vi "Reset Acyclic Channels.vi"(8 "error in (no error)":errorcluster, 11 "Single Board Loopback in":refnum<class "Single Board Loopback.lvclass">) -> (0 "error out":errorcluster, 3 "Single Board Loopback out":refnum<class "Single Board Loopback.lvclass">)   [LabVIEW 2020]
uses:
  Single Board Loopback/Single Board Loopback.lvclass
  C:/Users/nitest/Desktop/Git 2020/niveristand-custom-device-testing-tools/VeriStandTestCase/VeriStandTestCase.lvclass
  1e32ca70-98be-4c49-9a55-e48adc1a34b6.vi
  <vilib>/NI VeriStand/Execution/Workspace/NI VeriStand - Set Multiple Channel Values.vi
  niveristand-custom-device-testing-tools/VeriStandTestUtilities/VeriStandTestUtilities.lvlib
  <vilib>/NI VeriStand/Execution/Workspace/NI_VS Workspace ExecutionAPI.lvlib
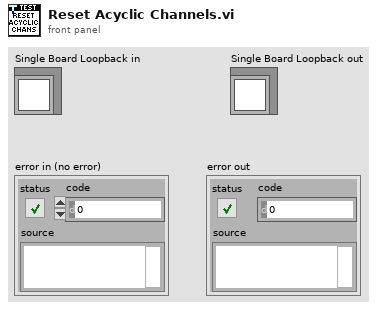
[diagram p1: front panel]
types:
  T1 = typedef "NI_VS Workspace ExecutionAPI.lvlib/WorkspaceAPI.ctl" = refnum<k24>
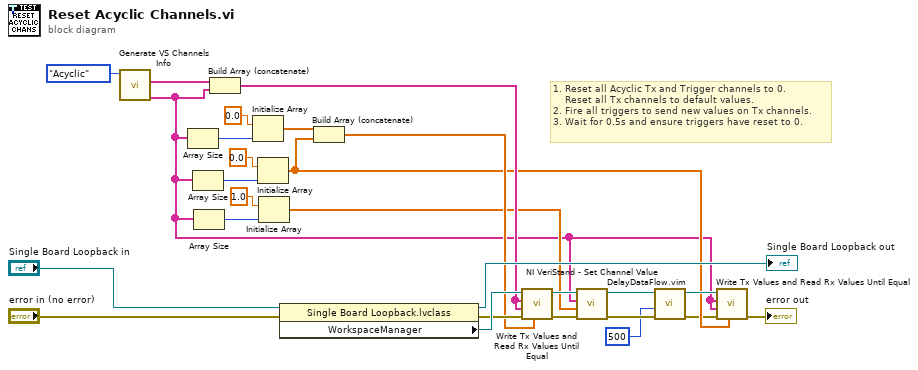
[diagram p0: block diagram]
diagram:
  # "1. Reset all Acyclic Tx and Trigger channels to 0.\n    Reset all Tx channels to default values.\n2. Fire all triggers to send new values on Tx channels.\n3. Wait for 0.5s and ensure triggers have reset to 0."
  n1 = call "Generate VS Channels Info.vi"("Transfer Type"=enum16{"Acyclic", "Scheduled"}."Acyclic") -> ("Tx Trigger Channels Array"=w1:string[], "Tx Channels Array"=w23:string[])  [unwired: 6 in, 3 out]
  n2 = Array Size(array=w1) -> (size(s)=w3:i32)
  n3 = Array Size(array=w1) -> (size(s)=w22:i32)
  n4 = Array Size(array=w1) -> (size(s)=w13:i32)
  n5 = Build Array (concatenate)(w23, w1) -> (w19:string[])
  n6 = Initialize Array(0.0 ("element"), w3) -> (w2:dbl[])
  n7 = Initialize Array(0.0 ("element"), w22) -> (w10:dbl[])
  n8 = Initialize Array(1.0 ("element"), w13) -> (w11:dbl[])
  n9 = property class="Single Board Loopback.lvclass"(reference="Single Board Loopback in", error in="error in (no error)") -> (reference out=→"Single Board Loopback out":refnum<class "Single Board Loopback.lvclass">, error out=w20:errorcluster, "WorkspaceManager"=w24:T1)
  n10 = Build Array (concatenate)(w2, w10) -> (w18:dbl[])
  n11 = call "Write Tx Values and Read Rx Values Until Equal.vi"("Tx values"=w18, "error in"=w20, "Rx aliases"=w19, "Tx aliases"=w19, "workspace manager in"=w24) -> ("error out"=w17:errorcluster, "workspace manager out"=w16:T1)  [unwired: 4 in, 1 out]
  n12 = call-poly <vilib>:"NI VeriStand - Set Channel Value.vi"("error in (no error)"=w17, "Values"=w11, "Channels"=w1, "WorkspaceManager in"=w16) -> ("error out"=w15:errorcluster, "WorkspaceManager out"=w14:T1)  [unwired: 6 in]
  n13 = call "DelayDataFlow.vim"("value in"=w15, "milliseconds to wait"=u32 500) -> ("value out"=w9:errorcluster)  [unwired: 2 in, 1 out]
  n14 = call "Write Tx Values and Read Rx Values Until Equal.vi"("Tx values"=w10, "error in"=w9, "Rx aliases"=w1, "Tx aliases"=w1, "workspace manager in"=w14) -> ("error out"=→"error out":errorcluster)  [unwired: 4 in, 2 out]
